vi "cblas dsyrk.vi"(0 "A":T4, 2 "C":T4, 3 "alpha":dbl=1.0, 4 "beta":dbl=1.0, 5 "order":T3=101 items=["CblasRowMajor"=101, "CblasColMajor"=102], 6 "transA":T1=111 items=["CblasNoTrans"=111, "CblasTrans"=112, "CblasConjTrans "=113], 7 "uplo":T2=121 items=["CblasUpper"=121, "CblasLower"=122], 8 "lda":i32, 11 "n":i32=-1, 12 "ldc":i32, 13 "k":i32=-1) -> (14 "dsyrk":T4, 19 "error":i32)   [LabVIEW 2020, in "NI_AALBLAS.lvlib"]
uses:
  <vilib>/Analysis/NI_AALBLAS.lvlib
  <vilib>/Analysis/Matrix/Datatypes/RealMatrix.ctl
  <vilib>/Analysis/BLAS.llb/Order.ctl
  <vilib>/Analysis/BLAS.llb/UpLo.ctl
  <vilib>/Analysis/BLAS.llb/Operation_Transpose.ctl
  <vilib>/Analysis/Matrix/NI_Matrix.lvlib
  <resource>/lvblas.dll
panel:
  # "void cblas_dsyrk(order, uplo, transA, n, k, alpha,*A, lda, beta, *C, ldc)"
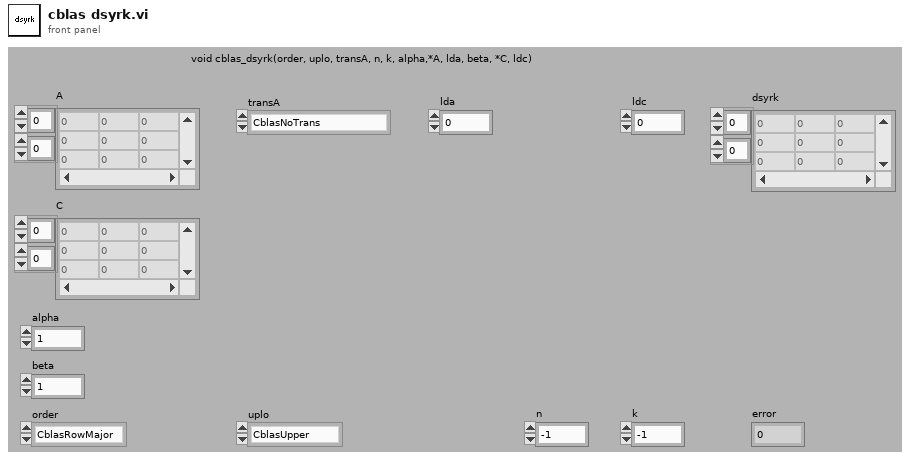
[diagram p1: front panel]
types:
  T1 = typedef "NI_AALBLAS.lvlib/Operation_Transpose.ctl" = i32
  T2 = typedef "NI_AALBLAS.lvlib/UpLo.ctl" = i32
  T3 = typedef "NI_AALBLAS.lvlib/Order.ctl" = i32
  T4 = typedef "NI_Matrix.lvlib/RealMatrix.ctl" = dbl[][]
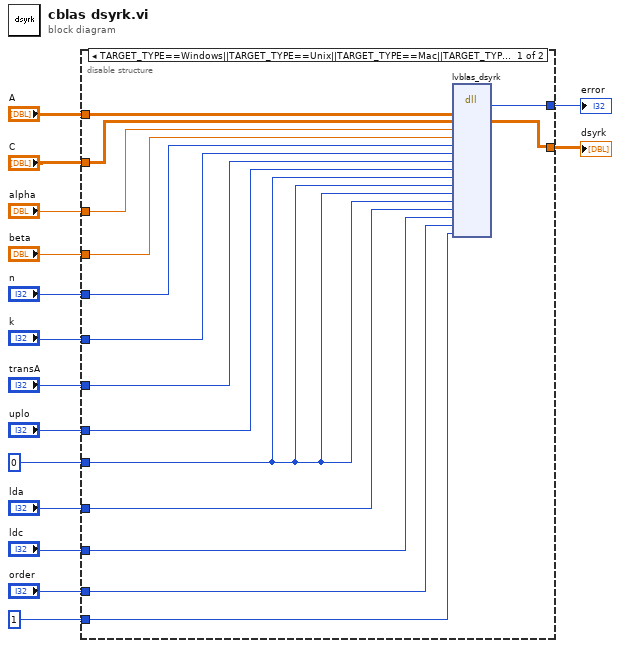
[diagram p0: block diagram]
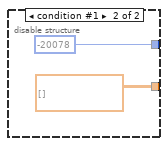
[diagram p2: hidden frame]
diagram:
  n1 = disable-structure shown="TARGET_TYPE==Windows||TARGET_TYPE==Unix||TARGET_TYPE==Mac||TARGET_TYPE==RT" {
    disable-tunnel: [w30 -20078 ("error")] -> w15
    disable-tunnel: "A" -> [w29 _]
    disable-tunnel: "C" -> [w28 _]
    disable-tunnel: "alpha" -> [w27 _]
    disable-tunnel: [w22 T4 [] ("Real Matrix")] -> w14
    disable-tunnel: "uplo" -> [w25 _]
    disable-tunnel: 0 -> [w23 _]
    disable-tunnel: "beta" -> [w26 _]
    disable-tunnel: "transA" -> [w24 _]
    disable-tunnel: "order" -> [w17 _]
    disable-tunnel: "lda" -> [w21 _]
    disable-tunnel: "ldc" -> [w20 _]
    disable-tunnel: "n" -> [w19 _]
    disable-tunnel: "k" -> [w18 _]
    disable-tunnel: 1 -> [w16 _]
    frame condition #0 (active) {
      n2 = dll-call lib="e:/builds/penguin/labview/branches/2020/dev/dist/resource/lvblas.*" fn="lvblas_dsyrk" ("CBLAS.dll:MtrxxMtrxH")("A"=w29, "C"=w28, "alpha"=w27, "beta"=w26, "n"=w19, "k"=w18, "trans"=w24, "uplo"=w25, "startARow"=w23, "startACol"=w23, "startCRow"=w23, "startCCol"=w23, "lda"=w21, "ldc"=w20, "order"=w17, "check"=w16) -> ("error"=w30:i32, "C"=w22:dbl[][])  [unwired: 18 in, 2 out]
    }
    frame condition #1 {
    }
  }
  "dsyrk" <- w14
  "error" <- w15
